vi "Build Low Priority Async.vi"(6 "Group":i32, 7 "Virtual Memory Unit in":refnum<class "Virtual Memory Unit.lvclass">, 8 "error in (no error)":errorcluster, 10 "Starting Address":u16 format="%04x", 11 "Major Frame in":refnum<class "Major Frame.lvclass">) -> (0 "error out":errorcluster, 2 "Next Available Address":u16 format="%04x", 3 "Major Frame out":refnum<class "Major Frame.lvclass">, 5 "Virtual Memory Unit out":refnum<class "Virtual Memory Unit.lvclass">)   [LabVIEW 2020, in "BCI-1553 API.lvlib" / "Major Frame.lvclass"]
doc: "Creates a single Low Priority Check, Execution, Configuration, and Data Field in memory.\n\nRequires 64 Registers for implementation. This is due to a slight difference in register offset."
uses:
  Major Frame.lvclass
  Dependencies/Virtual Memory Unit/Virtual Memory Unit.lvclass
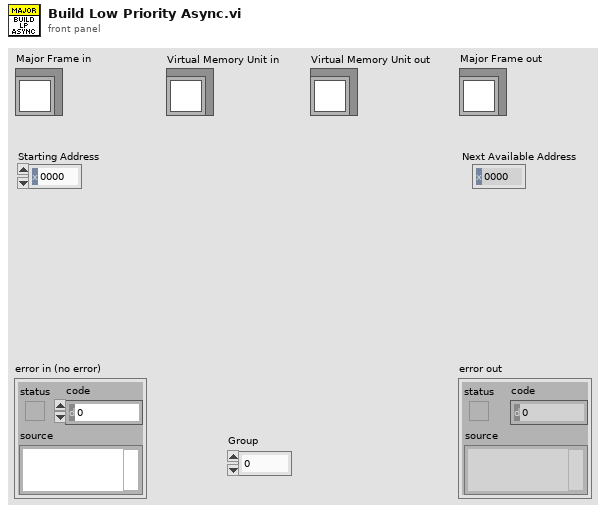
[diagram p1: front panel]
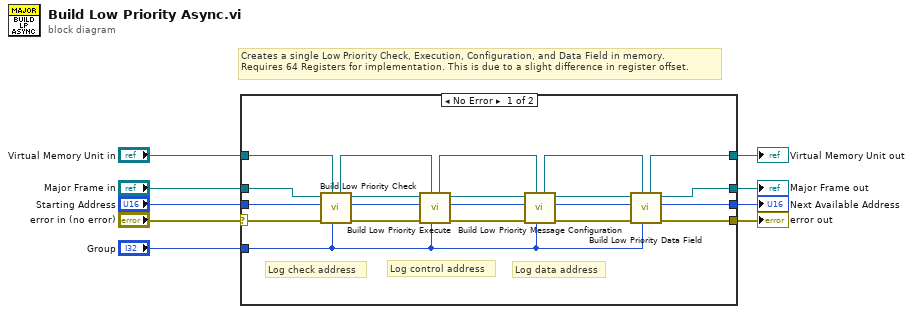
[diagram p0: block diagram]
diagram:
  # "Creates a single Low Priority Check, Execution, Configuration, and Data Field in memory.\nRequires 64 Registers for implementation. This is due to a slight difference in register offset."
  n1 = case shown="No Error" "error in (no error)" {
    selector: "error in (no error)" -> [w17 w33]
    tunnel: [w13 w33] -> w8
    tunnel: [w23 w32] -> w6
    tunnel: "Major Frame in" -> [w24 w32]
    tunnel: "Virtual Memory Unit in" -> [w22 w31]
    tunnel: [w18 w31] -> w4
    tunnel: "Starting Address" -> [w12 _]
    tunnel: "Group" -> [w11 _]
    tunnel: [w10 _] -> w1
    frame No Error {
      # "Log data address"
      # "Log control address"
      # "Log check address"
      n2 = call "Build Low Priority Check.vi"("Group"=w11, "Virtual Memory Unit in"=w22, "error in (no error)"=w17, "Starting Address"=w12, "Major Frame in"=w24) -> ("error out"=w16:errorcluster, "Next Available Address"=w27:u16, "Major Frame out"=w30:refnum<class "Major Frame.lvclass">, "Virtual Memory Unit out"=w21:refnum<class "Virtual Memory Unit.lvclass">)  [unwired: 3 in]
      n3 = call "Build Low Priority Execute.vi"("Group"=w11, "Virtual Memory Unit in"=w21, "error in (no error)"=w16, "Starting Address"=w27, "Major Frame in"=w30) -> ("error out"=w15:errorcluster, "Next Available Address"=w26:u16, "Major Frame out"=w29:refnum<class "Major Frame.lvclass">, "Virtual Memory Unit out"=w20:refnum<class "Virtual Memory Unit.lvclass">)  [unwired: 3 in]
      n4 = call "Build Low Priority Message Configuration.vi"("Group"=w11, "Virtual Memory Unit in"=w20, "error in (no error)"=w15, "Starting Address"=w26, "Major Frame in"=w29) -> ("error out"=w14:errorcluster, "Next Available Address"=w25:u16, "Major Frame out"=w28:refnum<class "Major Frame.lvclass">, "Virtual Memory Unit out"=w19:refnum<class "Virtual Memory Unit.lvclass">)  [unwired: 3 in]
      n5 = call "Build Low Priority Data Field.vi"("Group"=w11, "Virtual Memory Unit in"=w19, "error in (no error)"=w14, "Starting Address"=w25, "Major Frame in"=w28) -> ("error out"=w13:errorcluster, "Next Available Address"=w10:u16, "Major Frame out"=w23:refnum<class "Major Frame.lvclass">, "Virtual Memory Unit out"=w18:refnum<class "Virtual Memory Unit.lvclass">)  [unwired: 3 in]
    }
    frame Error {
    }
  }
  "error out" <- w8
  "Major Frame out" <- w6
  "Virtual Memory Unit out" <- w4
  "Next Available Address" <- w1
